vi "zad4.vi"() -> ()   [LabVIEW 2025]
panel:
  out "Gaussian noise pattern":dbl[](array[numeric])
  in  "Amp":dbl
  in  "phase":dbl
  in  "Sygnal":T1(ring)
  in  "liczba cykli":i64
  in  "samples":i32=128
  out "Waveform Chart":dbl[](graph)
  out "RMS":dbl
  out "kw":dbl
  out "arytm":dbl
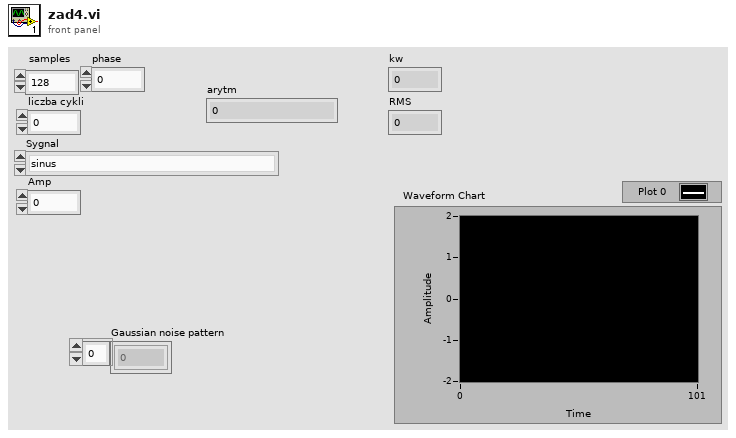
[diagram p1: front panel]
types:
  T1 = enum16{"sinus", "prostokat", "pila", "trojkat", "rozklad losowy", "rozklad normalny"}
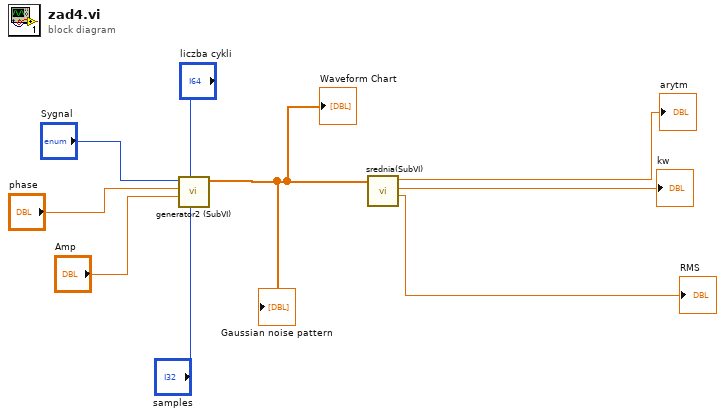
[diagram p0: block diagram]
diagram:
  n1 = call "generator2 (SubVI).vi"("samples"="samples", "liczba cykli"="liczba cykli", "Amp"="Amp", "phase"="phase", "Sygnal"="Sygnal") -> ("Gaussian noise pattern"=w1:dbl[])  [unwired: 6 in]
  "Waveform Chart" <- w1
  "Gaussian noise pattern" <- w1
  n2 = call "srednia(SubVI).vi"("input"=w1) -> ("RMS"=→"RMS":dbl, "kw"=→"kw":dbl, "arytm"=→"arytm":dbl)  [unwired: 8 in]
